vi "Create TDMS Channels - XNET CAN.vi"(5 "XNET Cluster":refnum<k21>="ManyXnetChannels", 7 "CAN Interface":refnum<k21>="CAN1", 8 "error in (no error)":errorcluster, 10 "group name in":string="Log", 11 "TDMS ref in":refnum<k34>) -> (0 "error out":errorcluster, 1 "Signal Names":string[](array[string]), 2 "group name out":string="Log", 3 "TDMS ref out":refnum<k34>, 4 "Signal Units":string[](array[string]))   [LabVIEW 2021, in "XNET-CAN-Signal-Logger.lvlib"]
uses:
  XNET-CAN-Signal-Logger.lvlib
  <resource>/objmgr/xnet.rc
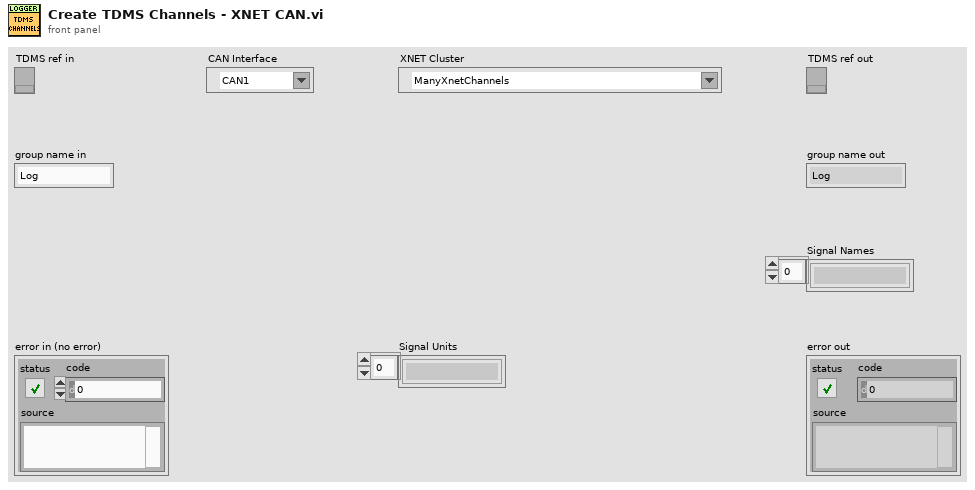
[diagram p1: front panel]
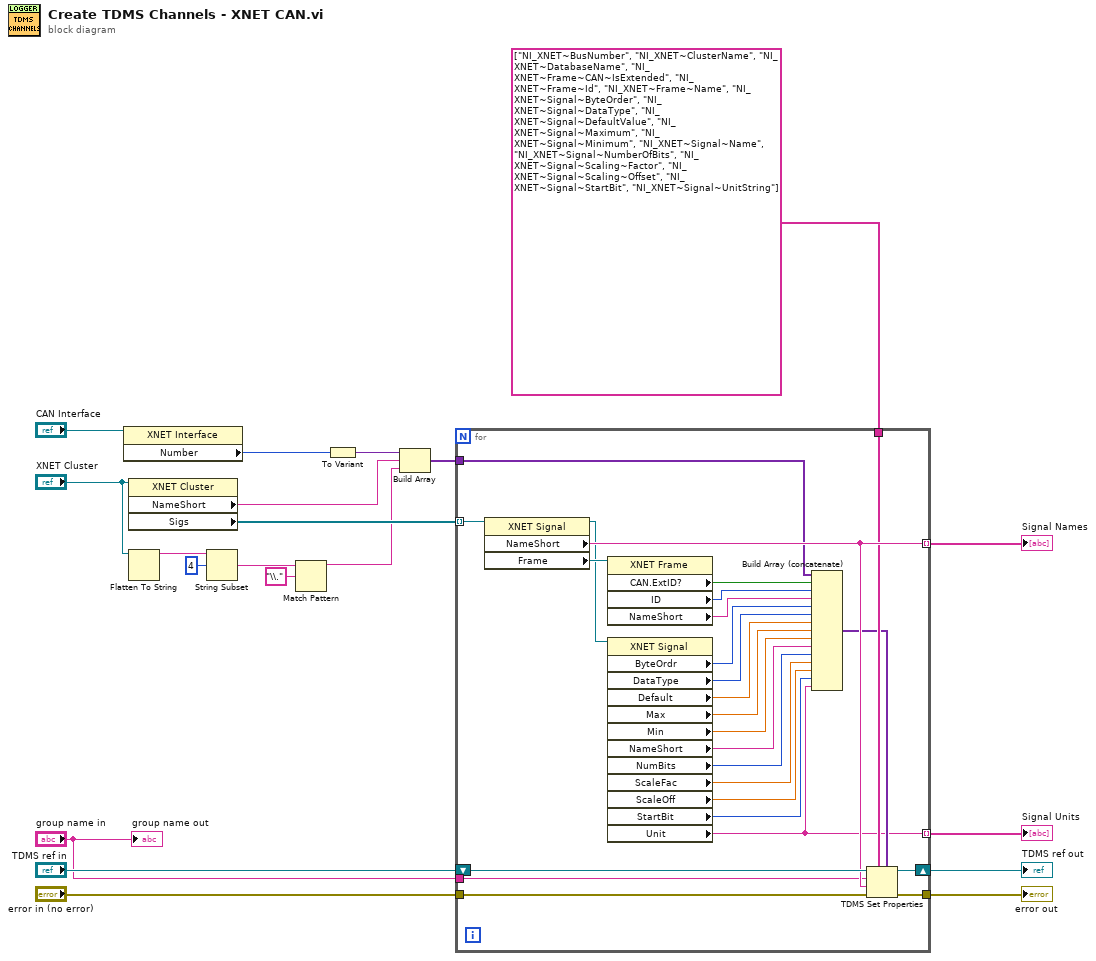
[diagram p0: block diagram]
diagram:
  n1 = property class="XNET Interface"(reference="CAN Interface") -> ("Number"=w11:u32)  [unwired: 1 in, 2 out]
  n2 = property class="XNET Cluster"(reference="XNET Cluster") -> ("NameShort"=w4:string, "Sigs"=w8:refnum<k21>[])  [unwired: 1 in, 2 out]
  n3 = Flatten To String(anything="XNET Cluster") -> (data string=w13:string)  [unwired: 3 in, 2 out]
  n4 = String Subset(string=w13, offset (0)=4) -> (substring=w9:string)  [unwired: 1 in]
  n5 = Match Pattern(string=w9, regular expression="\\.") -> (before substring=w2:string)  [unwired: 1 in, 3 out]
  n6 = To Variant(anything=w11) -> (Variant=w10:variant)
  n7 = Build Array(w10, w4, w2) -> (w7:variant[])
  n8 = for {
    tunnel: w8 -> [w46] mode=indexing
    tunnel: [w44] -> w16 mode=indexing
    shift-right: [w42] -> w18
    shift-left: "TDMS ref in" -> [w45]
    tunnel: "error in (no error)" -> [w43]
    tunnel: [w41] -> w20
    tunnel: string[] ["NI_XNET~BusNumber", "NI_XNET~ClusterName", "NI_XNET~DatabaseName", "NI_XNET~Frame~CAN~IsExtended", "NI_XNET~Frame~Id", "NI_XNET~Frame~Name", "NI_XNET~Signal~ByteOrder", "NI_XNET~Signal~DataType", "NI_XNET~Signal~DefaultValue", "NI_XNET~Signal~Maximum", "NI_XNET~Signal~Minimum", "NI_XNET~Signal~Name", "NI_XNET~Signal~NumberOfBits", "NI_XNET~Signal~Scaling~Factor", "NI_XNET~Signal~Scaling~Offset", "NI_XNET~Signal~StartBit", "NI_XNET~Signal~UnitString"] ("property names") -> [w40]
    tunnel: w7 -> [w37]
    tunnel: "group name in" -> [w22]
    tunnel: [w21] -> w5 mode=indexing
    n9 = property class="XNET Signal"(reference=w46) -> (reference out=w38:refnum<k21>, "NameShort"=w44:string, "Frame"=w39:refnum<k21>)  [unwired: 1 in, 1 out]
    n10 = property class="XNET Frame"(reference=w39) -> ("CAN.ExtID?"=w35:bool, "ID"=w34:u32, "NameShort"=w33:string)  [unwired: 1 in, 2 out]
    n11 = property class="XNET Signal"(reference=w38) -> ("ByteOrdr"=w32:u32, "DataType"=w31:u32, "Default"=w30:dbl, "Max"=w29:dbl, "Min"=w28:dbl, "NameShort"=w27:string, "NumBits"=w26:u32, "ScaleFac"=w25:dbl, "ScaleOff"=w24:dbl, "StartBit"=w23:u32, "Unit"=w21:string)  [unwired: 1 in, 2 out]
    n12 = Build Array (concatenate)(w37, w35, w34, w33, w32, w31, w30, w29, w28, w27, w26, w25, w24, w23, w21) -> (w36:variant[])
    n13 = TDMS Set Properties(5:w36, 7:w40, 8:w43, 9:w44, 10:w22, 11:w45) -> (0:w41:errorcluster, 3:w42:refnum<k34>)  [unwired: 2 out]
  }
  "error out" <- w20
  "TDMS ref out" <- w18
  "Signal Names" <- w16
  "Signal Units" <- w5
  "group name out" <- "group name in"
